vi "Mandelbro_display.vi"() -> ()   [LabVIEW 2015]
uses:
  time_logic.vi
panel:
  out "error out":errorcluster
  in  "Ip":string
  in  "stop":bool
  out "Throughput":dbl(graph)
  out "VARIANT IN CASE OF ERROR":variant
  in  "Reset Picture":bool
  out "Errors":i32
  out "XY Graph":cluster{"X":dbl, "Y":dbl}[](graph)
  out "Data Read":i32
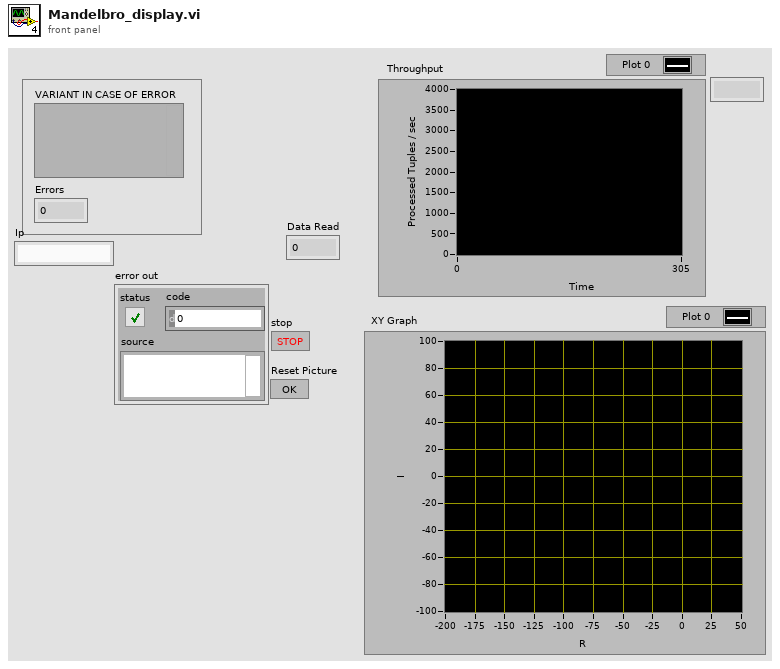
[diagram p1: front panel]
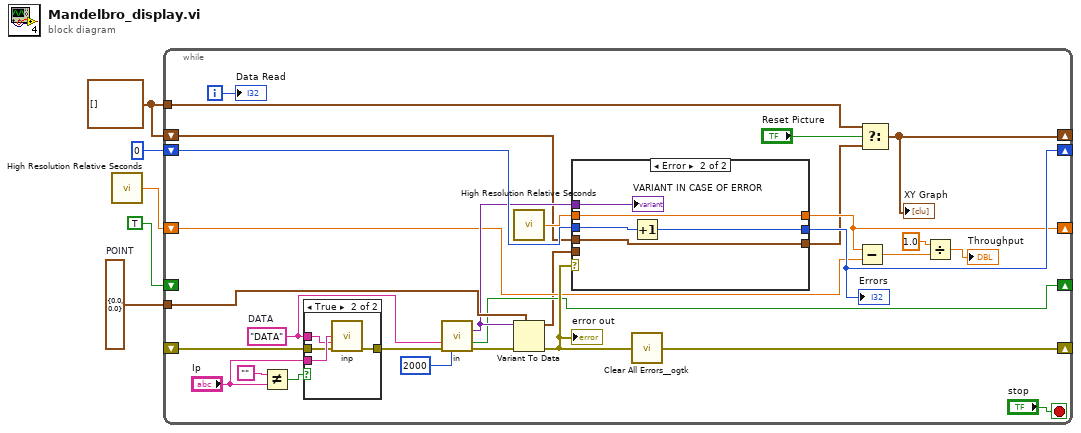
[diagram p0: block diagram]
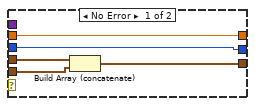
[diagram p3: hidden frame]
diagram:
  w3 = cluster{"X":dbl, "Y":dbl}[] []
  w5 = cluster{"X":dbl, "Y":dbl} {"X"=0.0, "Y"=0.0}  # POINT
  n1 = call <vilib>:"High Resolution Relative Seconds.vi"() -> ("relative seconds"=w2:dbl)
  n2 = while {
    tunnel: w5 -> [w32]
    shift-right: [w10] -> _
    shift-left: w3 -> [w7]
    shift-right: [w31] -> _
    shift-left: _ -> [w12]
    shift-right: [w28] -> _
    shift-left: 0 -> [w29]
    tunnel: w3 -> [w27]
    shift-right: [w23] -> _
    shift-left: w2 -> [w24]
    shift-right: [w19] -> _
    shift-left: TRUE ("Valid data") -> [_]
    i -> [w33]
    stop <- "stop" stop-if-true
    w14 = "DATA"  # DATA
    n3 = Not Equal?(x="", y="Ip") -> (x != y?=w13:bool)
    n4 = case shown="True" w13 {
      tunnel: "Ip" -> [_ w39]
      tunnel: w14 -> [_ w38]
      tunnel: w12 -> [w35 w37]
      tunnel: [w35 w36] -> w11
      frame False {
      }
      frame True {
        n5 = call "inp.vi"("Ip"=w39, "Name in"=w38, "error in (no error)"=w37) -> ("error out"=w36:errorcluster)  [unwired: 10 in, 2 out]
      }
    }
    n6 = call "in.vi"("Name in"=w14, "error in (no error)"=w11, "timout"=2000) -> ("OUT VARIANT"=w25:variant, "Valid data"=w19:bool, "error out"=w34:errorcluster)  [unwired: 10 in]
    n7 = call <vilib>:"High Resolution Relative Seconds.vi"() -> ("relative seconds"=w18:dbl)
    n8 = Variant To Data(error in=w34, type=w32, Variant=w25) -> (data=w8:cluster{"X":dbl, "Y":dbl}, error out=w30:errorcluster)
    "error out" <- w30
    n9 = case shown="Error" w30 {
      tunnel: w29 -> [w44 w49]
      tunnel: [w44 w48] -> w28
      tunnel: w25 -> [_ w47]
      tunnel: [w43 w46] -> w23
      tunnel: w18 -> [w43 w46]
      tunnel: w8 -> [w42 _]
      tunnel: w7 -> [w41 w45]
      tunnel: [w40 w45] -> w6
      frame No Error {
        n10 = Build Array (concatenate)(w41, w42) -> (w40:cluster{"X":dbl, "Y":dbl}[])
      }
      frame Error {
        n11 = Increment(x=w49) -> (x+1=w48:i32)
        "VARIANT IN CASE OF ERROR" <- w47
      }
    }
    "Errors" <- w28
    n12 = call <userlib>:"Clear All Errors__ogtk.vi"("Error In"=w30) -> ("Error Out"=w31:errorcluster)  [unwired: 3 in]
    n13 = Subtract(x=w23, y=w24) -> (x-y=w21:dbl)
    n14 = Select(t=w27, s="Reset Picture", f=w6) -> (s? t:f=w10:cluster{"X":dbl, "Y":dbl}[])
    "XY Graph" <- w10
    n15 = Divide(x=1.0, y=w21) -> (x/y=→"Throughput":dbl)
    "Data Read" <- w33
  }
